vi "Create Document.vi"(8 "error in (no error)":errorcluster, 10 "Root Element Name (\"\" = none)":string) -> (0 "error out":errorcluster, 2 "Root Element":refnum<k20>, 3 "Document":refnum<k20>)   [LabVIEW 2013, in "JUnit XML.lvlib"]
doc: "Creates a new document with the specified root element. The caller is responsible for cleaning up references."
uses:
  JUnit XML.lvlib
  <vilib>/xml/NI_XML.lvlib
  <resource>/objmgr/DOMUserDefRef.rc
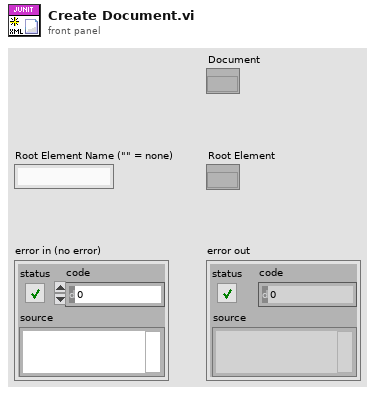
[diagram p1: front panel]
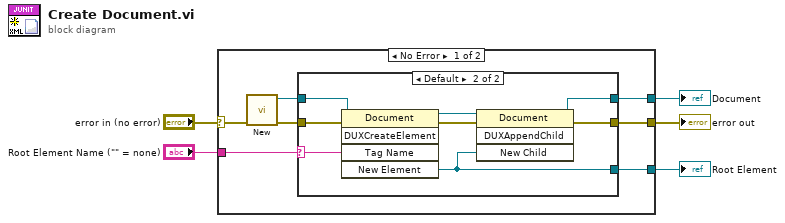
[diagram p0: block diagram]
diagram:
  n1 = case shown="No Error" "error in (no error)" {
    selector: "error in (no error)" -> [w7 w23]
    tunnel: "Root Element Name (\"\" = none)" -> [w6 _]
    tunnel: [w11 _] -> w4
    tunnel: [w9 w23] -> w3
    tunnel: [w8 _] -> w2
    frame No Error {
      n2 = call <vilib>:"New.vi"("error in (no error)"=w7) -> ("error out"=w12:errorcluster, "DOM document out"=w10:refnum<k20>)  [unwired: 7 in]
      n3 = case shown="Default" w6 {
        selector: w6 -> [_ w15]
        tunnel: w12 -> [w13 w22]
        tunnel: [_ w19] -> w11
        tunnel: w10 -> [w14 w18]
        tunnel: [w13 w17] -> w9
        tunnel: [w14 w16] -> w8
        frame "\u0000" {
        }
        frame Default {
          n4 = invoke class="Document" method="DUXCreateElement"(reference=w18, error in=w22, "Tag Name"=w15) -> (reference out=w20:refnum<k20>, error out=w21:errorcluster, "New Element"=w19:refnum<k20>)  [unwired: 2 in, 2 out]
          n5 = invoke class="Document" method="DUXAppendChild"(reference=w20, error in=w21, "New Child"=w19) -> (reference out=w16:refnum<k20>, error out=w17:errorcluster)  [unwired: 1 in, 2 out]
        }
      }
    }
    frame Error {
    }
  }
  "error out" <- w3
  "Document" <- w2
  "Root Element" <- w4
